vi "Global.vi"() -> ()   [LabVIEW 2020]
panel:
  in  "判定长度":i32
  in  "上序状态":refnum<vi>
  in  "CODE_ID":string
  out "启用第二段":bool
  in  "第一段判定参数":T1
  in  "结果判定参数":T2
  in  "判定框参数":T3
  in  "USER_ID":string
  in  "DEVICED_ID":string
  in  "FRE_ID":string
  in  "PRODUCT_ID":string
  in  "合格数量":i32
  in  "生产数量":i32
  in  "试验项目":bool[](array[boolean])
  out "模式":u32
  in  "更换产品":refnum<vi>
  in  "提示信息":refnum<vi>
  in  "程序自动":refnum<vi>
  in  "报警图标":refnum<vi>
  in  "程序关闭":bool
  in  "Info":refnum<vi>
  in  "Result":refnum<vi>
  in  "批次":refnum<vi>
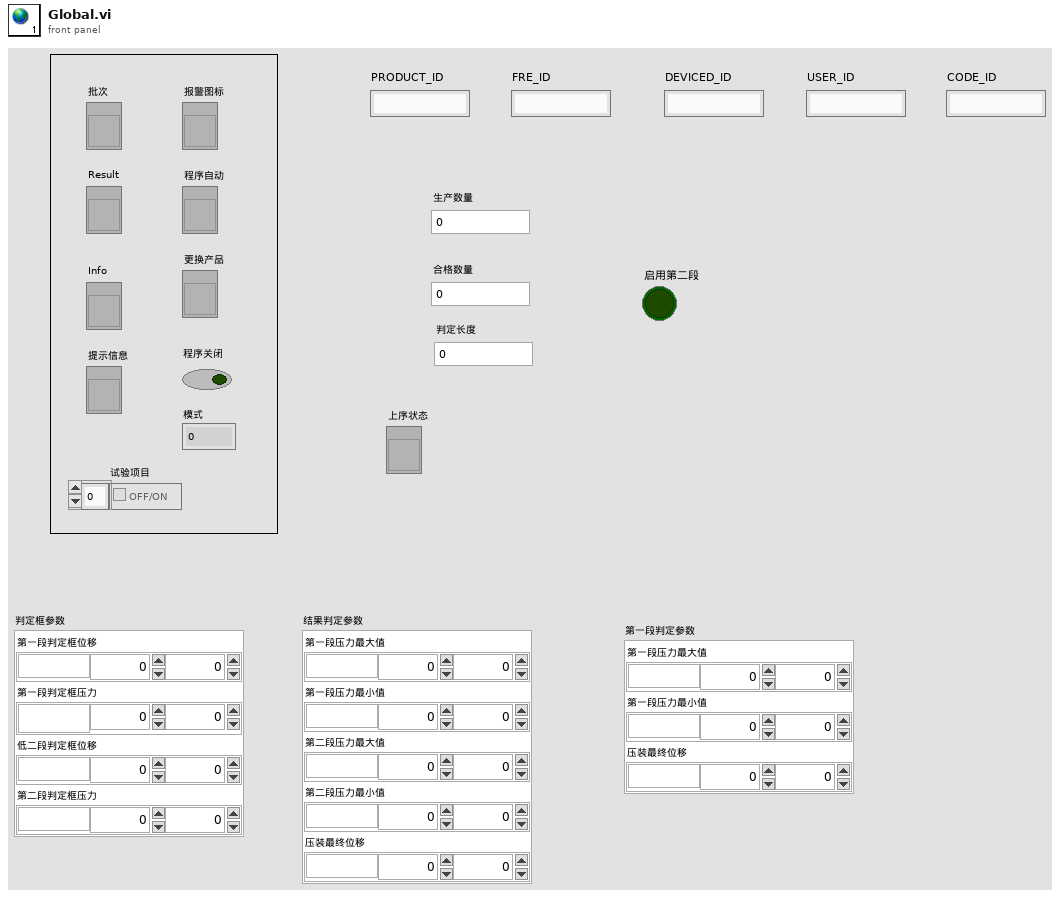
[diagram p1: front panel]
types:
  T1 = cluster{"第一段压力最大值":cluster{"单位":string, "下限":dbl, "上限":dbl}, "第一段压力最小值":cluster{"单位":string, "下限":dbl, "上限":dbl}, "压装最终位移":cluster{"单位":string, "下限":dbl, "上限":dbl}}
  T2 = cluster{"第一段压力最大值":cluster{"单位":string, "下限":dbl, "上限":dbl}, "第一段压力最小值":cluster{"单位":string, "下限":dbl, "上限":dbl}, "第二段压力最大值":cluster{"单位":string, "下限":dbl, "上限":dbl}, "第二段压力最小值":cluster{"单位":string, "下限":dbl, "上限":dbl}, "压装最终位移":cluster{"单位":string, "下限":dbl, "上限":dbl}}
  T3 = cluster{"第一段判定框位移":cluster{"单位":string, "下限":dbl, "上限":dbl}, "第一段判定框压力":cluster{"单位":string, "下限":dbl, "上限":dbl}, "低二段判定框位移":cluster{"单位":string, "下限":dbl, "上限":dbl}, "第二段判定框压力":cluster{"单位":string, "下限":dbl, "上限":dbl}}
diagram:
